vi "SMO.Example.VI Tree.vi"() -> ()   [LabVIEW 2013, in "SMO.Example.lvclass"]
uses:
  SMO.Example.lvclass
  Typedefs/DataChanged--EventData--Cluster.ctl
  Typedefs/PrivateData--Cluster.ctl
  Typedefs/Configuration--Cluster.ctl
  Typedefs/PublicEvents--Cluster.ctl
  Typedefs/ProtectedEvents--Cluster.ctl
  Typedefs/API Inputs--Cluster.ctl
  Typedefs/PumpState--Cluster.ctl
  Typedefs/ValveState--Cluster.ctl
  SMO/SMO.lvclass
panel:
  in  "SMO.Example":refnum<class "SMO.Example.lvclass">
  in  "Public Events":T1
  in  "Configuration":T2
  in  "Private Data":T3
  in  "Data In Event Data":T5
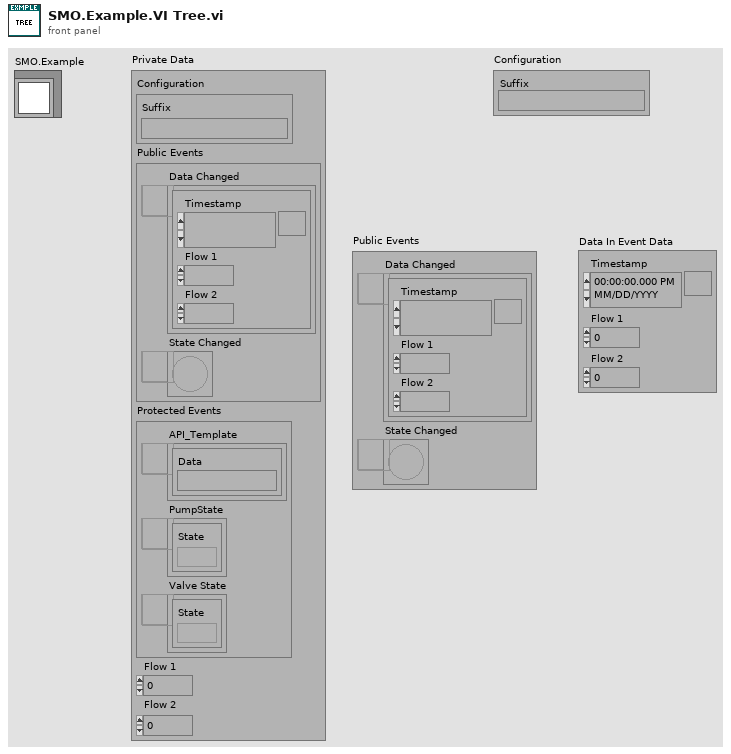
[diagram p1: front panel]
types:
  T1 = typedef "SMO.Example.lvclass/PublicEvents--Cluster.ctl" = cluster{"Data Changed":refnum<user-event>, "State Changed":refnum<user-event>}
  T2 = typedef "SMO.Example.lvclass/Configuration--Cluster.ctl" = cluster{"Suffix":string}
  T3 = typedef "SMO.Example.lvclass/PrivateData--Cluster.ctl" = cluster{"Configuration":T2, "Public Events":T1, "Protected Events":T4, "Flow 1":dbl, "Flow 2":dbl}
  T4 = typedef "SMO.Example.lvclass/ProtectedEvents--Cluster.ctl" = cluster{"API_Template":refnum<user-event>, "PumpState":refnum<user-event>, "Valve State":refnum<user-event>}
  T5 = typedef "SMO.Example.lvclass/DataChanged--EventData--Cluster.ctl" = cluster{"Timestamp":timestamp, "Flow 1":dbl, "Flow 2":dbl}
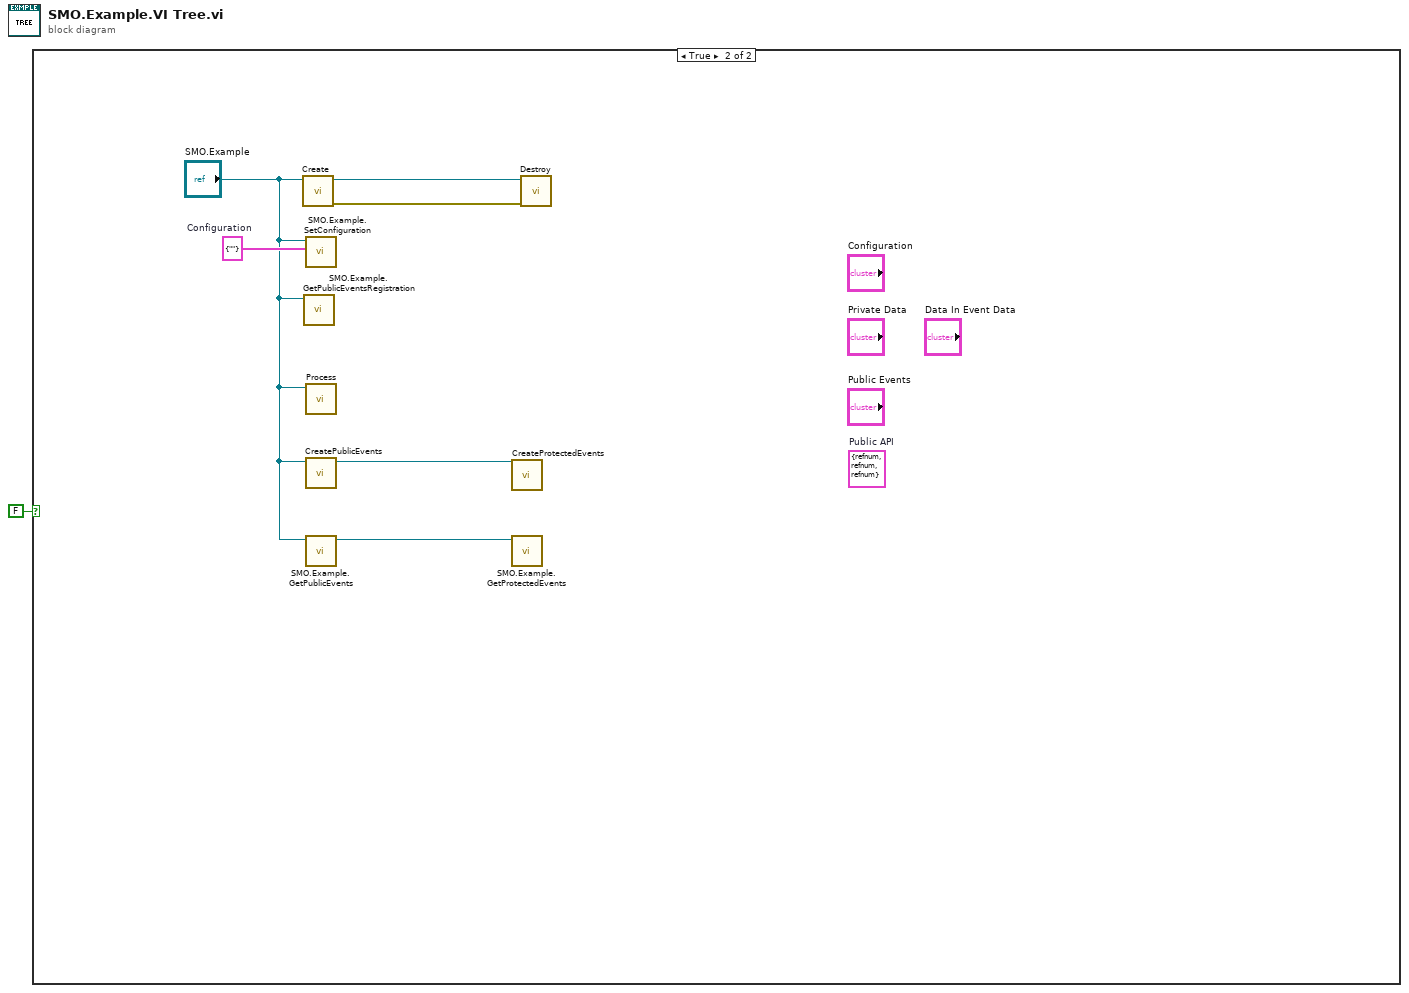
[diagram p0: block diagram]
diagram:
  n1 = case shown="True" FALSE {
    frame False {
    }
    frame True {
      (unwired) T4 {"API_Template"=refnum, "PumpState"=refnum, "Valve State"=refnum}  # Public API
      w7 = T2 {"Suffix"=""}  # Configuration
      n2 = call "Create.vi"("SMO"="SMO.Example") -> ("error out"=w4:errorcluster, "SMO out"=w5:refnum<class "SMO.Example.lvclass">)  [unwired: 8 in, 1 out]
      n3 = call "SMO.Example.GetPublicEventsRegistration.vi"("SMO.Example"="SMO.Example") -> ()  [unwired: 8 in, 3 out]
      n4 = call "SMO.Example.SetConfiguration.vi"("Configuration"=w7, "SMO.Example"="SMO.Example") -> ()  [unwired: 8 in, 2 out]
      n5 = call-dynamic "Process.vi"("SMO.Example"="SMO.Example") -> ()  [unwired: 9 in, 2 out]
      n6 = call-dynamic "CreatePublicEvents.vi"("SMO.Example"="SMO.Example") -> ("SMO.Example out"=w2:refnum<class "SMO.Example.lvclass">)  [unwired: 9 in, 1 out]
      n7 = call "SMO.Example.GetPublicEvents.vi"("SMO.Example"="SMO.Example") -> ("SMO.Example out"=w6:refnum<class "SMO.Example.lvclass">)  [unwired: 8 in, 2 out]
      n8 = call-dynamic "CreateProtectedEvents.vi"("JKI SMO.Example"=w2) -> ()  [unwired: 9 in, 2 out]
      n9 = call "SMO.Example.GetProtectedEvents.vi"("SMO.Example"=w6) -> ()  [unwired: 8 in, 3 out]
      n10 = call "Destroy.vi"("error in (no error)"=w4, "SMO"=w5) -> ()  [unwired: 9 in, 1 out]
    }
  }
